vi "校准时拍照自动存图-Cam1夹角校准.vi"(9 "左边图/右边图":enum16{"左边", "右边"}(ring), 11 "Img输入":T1) -> ()   [LabVIEW 2014]
uses:
  <vilib>/vision/Image Controls.llb/IMAQ Image.ctl
  Global.vi
panel:
  out "添加的路径":path
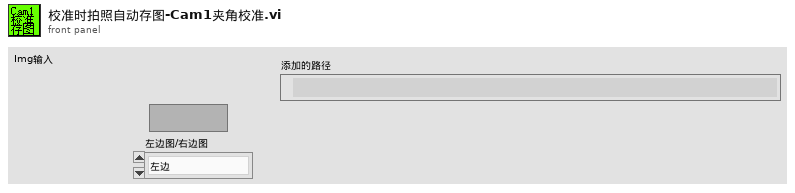
[diagram p1: front panel]
types:
  T1 = typedef "IMAQ Image.ctl" = refnum<image>
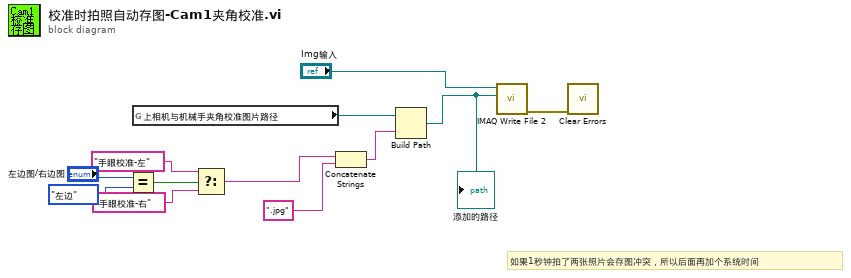
[diagram p0: block diagram]
diagram:
  # "如果1秒钟拍了两张照片会存图冲突，所以后面再加个系统时间"
  n1 = Equal?(x="左边图/右边图", y=enum16{"左边", "右边"}."左边") -> (x = y?=w4:bool)
  n2 = global read "Global.vi" "上相机与机械手夹角校准图片路径"() -> (w11:path)
  n3 = Select(t="手眼校准-左" ("字符串"), s=w4, f="手眼校准-右" ("字符串")) -> (s? t:f=w1:string)
  n4 = Concatenate Strings(w1, ".jpg" ("字符串")) -> (w9:string)
  n5 = Build Path(base path=w11, name or relative path=w9) -> (appended path=w10:path)
  "添加的路径" <- w10
  n6 = call-poly "IMAQ Write File 2"("File Path"=w10, "Image"="Img输入") -> ("error out"=w8:errorcluster)  [unwired: 8 in, 1 out]
  n7 = call <vilib>:"Clear Errors.vi"("error in (no error)"=w8) -> ()  [unwired: 5 in, 2 out]
